vi "16转2进制字符串.vi"(1 "16进制字符串":string) -> (0 "转换后二进制字符":string)   [LabVIEW 2018]
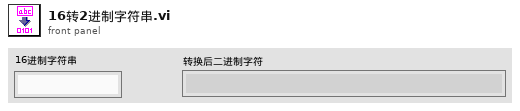
[diagram p1: front panel]
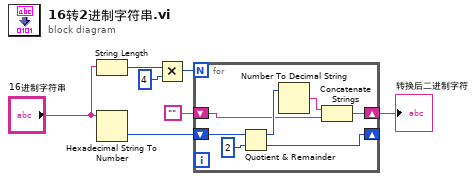
[diagram p0: block diagram]
diagram:
  n1 = String Length(string="16进制字符串") -> (length=w4:i32)
  n2 = Hexadecimal String To Number(string="16进制字符串") -> (number=w6:u32)  [unwired: 2 in, 1 out]
  n3 = Multiply(x=w4, y=4) -> (x*y=w2:i32)
  n4 = for {
    N: w2 -> [_]
    shift-right: [w14] -> w1
    shift-left: "" -> [w9]
    shift-right: [w11] -> _
    shift-left: w6 -> [w10]
    n5 = Quotient & Remainder(x=w10, y=2) -> (x-y*floor(x/y)=w12:u32, floor(x/y)=w11:u32)
    n6 = Number To Decimal String(number=w12) -> (decimal integer string=w8:string)  [unwired: 1 in]
    n7 = Concatenate Strings(w8, w9) -> (w14:string)
  }
  "转换后二进制字符" <- w1
